vi "Synchronise_Console_PC.vi"() -> (0 "PC_time = Console_time?":bool)   [LabVIEW 2013]
uses:
  VantagePro.dll
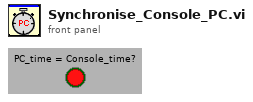
[diagram p1: front panel]
types:
  T1 = typedef "LVDateTimeRec.ctl" = cluster{"fractional second":dbl, "second":i32, "minute":i32, "hour":i32, "day of month":i32, "month":i32, "year":i32, "day of week":i32, "day of year":i32, "DST":i32}
  T2 = cluster{"minute":i32, "hour":i32, "day of month":i32, "month":i32, "year":i32}
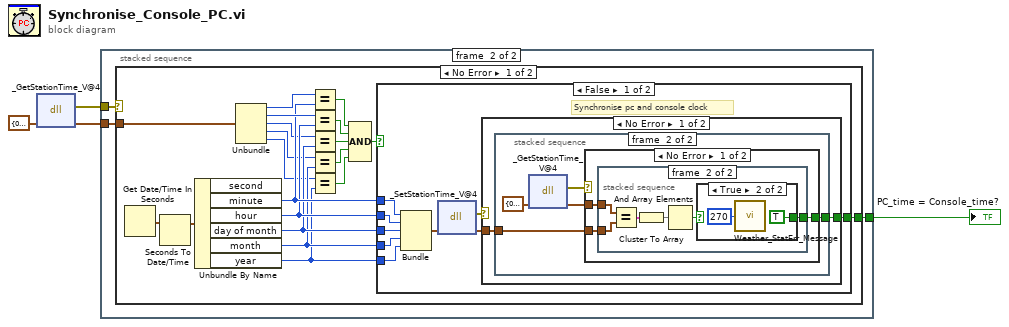
[diagram p0: block diagram]
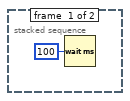
[diagram p2: hidden frame]
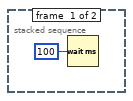
[diagram p3: hidden frame]
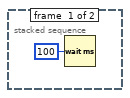
[diagram p4: hidden frame]
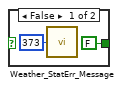
[diagram p5: hidden frame]
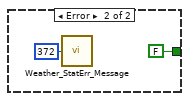
[diagram p6: hidden frame]
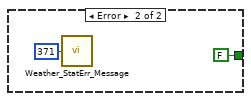
[diagram p7: hidden frame]
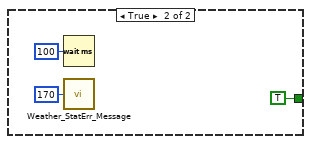
[diagram p8: hidden frame]
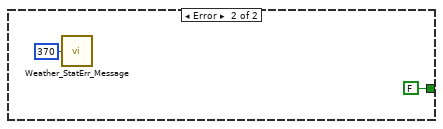
[diagram p9: hidden frame]
diagram:
  n1 = dll-call lib="C:/Users/vaneijk/Documents/LabView Projects 13/HiSPARC Weather Station/Develop/VantagePro.dll" fn="_GetStationTime_V@4" label="Get station time"("WeatherUnits"=cluster{i32, i32, i32, i32, i32} {0, 0, 0, 0, 0} ("Original Console time")) -> (error out=w2:errorcluster, "WeatherUnits"=w4:cluster{i32, i32, i32, i32, i32})  [unwired: 3 in, 2 out]
  n2 = stacked-sequence {
    tunnel: w4 -> [_ w8]
    tunnel: w2 -> [_ w7]
    tunnel: [_ w6] -> w1
    frame #0 {
      n3 = Wait (ms)(milliseconds to wait=u32 100) -> ()  [unwired: 1 out]
    }
    frame #1 {
      n4 = case shown="No Error" w7 {
        tunnel: w8 -> [w26 _]
        tunnel: [w21 FALSE] -> w6
        frame No Error {
          n5 = Get Date/Time In Seconds() -> (seconds since 1Jan1904=w28:timestamp)
          n6 = Seconds To Date/Time(time stamp (now)=w28) -> (date time rec=w27:T1)  [unwired: 1 in]
          n7 = Unbundle By Name(w27) -> ("minute"=w23:i32, "hour"=w22:i32, "day of month"=w20:i32, "month"=w19:i32, "year"=w18:i32)  [unwired: 1 out]
          n8 = Unbundle(w26) -> (w25:i32, w24:i32, w12:i32, w11:i32, w10:i32)
          n9 = Equal?(x=w25, y=w23) -> (x = y?=w17:bool)
          n10 = Equal?(x=w24, y=w22) -> (x = y?=w14:bool)
          n11 = Equal?(x=w12, y=w20) -> (x = y?=w13:bool)
          n12 = Equal?(x=w11, y=w19) -> (x = y?=w15:bool)
          n13 = Equal?(x=w10, y=w18) -> (x = y?=w16:bool)
          n14 = Compound Arithmetic op=AND(w17, w14, w13, w15, w16) -> (w9:bool)
          n15 = case shown="False" w9 {
            tunnel: w18 -> [w32 _]
            tunnel: w19 -> [w33 _]
            tunnel: w20 -> [w34 _]
            tunnel: w22 -> [w35 _]
            tunnel: w23 -> [w36 _]
            tunnel: [w29 TRUE] -> w21
            frame False {
              # "Synchronise pc and console clock"
              n16 = Bundle("minute"=w36, "hour"=w35, "day of month"=w34, "month"=w33, "year"=w32) -> (w37:T2)  [unwired: 1 in]
              n17 = dll-call lib="C:/Users/vaneijk/Documents/LabView Projects 13/HiSPARC Weather Station/Develop/VantagePro.dll" fn="_SetStationTime_V@4" label="Set station time"("dateTime"=w37) -> (error out=w31:errorcluster, "dateTime"=w30:T2)  [unwired: 3 in, 2 out]
              n18 = case shown="No Error" w31 {
                tunnel: w30 -> [w39 _]
                tunnel: [w38 FALSE] -> w29
                frame No Error {
                  n19 = stacked-sequence {
                    tunnel: w39 -> [_ w42]
                    tunnel: [_ w41] -> w38
                    frame #0 {
                      n20 = Wait (ms)(milliseconds to wait=u32 100) -> ()  [unwired: 1 out]
                    }
                    frame #1 {
                      n21 = dll-call lib="C:/Users/vaneijk/Documents/LabView Projects 13/HiSPARC Weather Station/Develop/VantagePro.dll" fn="_GetStationTime_V@4" label="Get station time"("WeatherUnits"=cluster{i32, i32, i32, i32, i32} {0, 0, 0, 0, 0}) -> (error out=w44:errorcluster, "WeatherUnits"=w43:cluster{i32, i32, i32, i32, i32})  [unwired: 3 in, 2 out]
                      n22 = case shown="No Error" w44 {
                        tunnel: w43 -> [w48 _]
                        tunnel: w42 -> [w47 _]
                        tunnel: [w46 FALSE] -> w41
                        frame No Error {
                          n23 = stacked-sequence {
                            tunnel: w47 -> [_ w55]
                            tunnel: w48 -> [_ w54]
                            tunnel: [_ w50] -> w46
                            frame #0 {
                              n24 = Wait (ms)(milliseconds to wait=u32 100) -> ()  [unwired: 1 out]
                            }
                            frame #1 {
                              n25 = Equal?(x=w54, y=w55) -> (x = y?=w53:cluster{bool, bool, bool, bool, bool})
                              n26 = Cluster To Array(cluster=w53) -> (array=w52:bool[])
                              n27 = And Array Elements(Boolean array=w52) -> (logical AND=w51:bool)
                              n28 = case shown="True" w51 {
                                tunnel: [FALSE TRUE] -> w50
                                frame False {
                                n29 = call "Weather_StatErr_Message.vi"("Message number"=373) -> ()  [unwired: 1 out]
                                }
                                frame True {
                                n30 = call "Weather_StatErr_Message.vi"("Message number"=270) -> ()  [unwired: 1 out]
                                }
                              }
                            }
                          }
                        }
                        frame Error {
                          n31 = call "Weather_StatErr_Message.vi"("Message number"=372) -> ()  [unwired: 1 out]
                        }
                      }
                    }
                  }
                }
                frame Error {
                  n32 = call "Weather_StatErr_Message.vi"("Message number"=371) -> ()  [unwired: 1 out]
                }
              }
            }
            frame True {
              n33 = Wait (ms)(milliseconds to wait=u32 100) -> ()  [unwired: 1 out]
              n34 = call "Weather_StatErr_Message.vi"("Message number"=170) -> ()  [unwired: 1 out]
            }
          }
        }
        frame Error {
          n35 = call "Weather_StatErr_Message.vi"("Message number"=370) -> ()  [unwired: 1 out]
        }
      }
    }
  }
  "PC_time = Console_time?" <- w1
